vi "Abort Panel VI.vi"(8 "error in (no error)":errorcluster, 11 "Console in":refnum<class "Console.lvclass">) -> (0 "error out":errorcluster, 3 "Console out":refnum<class "Console.lvclass">)   [LabVIEW 2015, in "EditPanel API.lvlib" / "Console.lvclass"]
uses:
  Console.lvclass
  Console.lvclass/Console.ctl
  Console Reply/Console Reply/Console Reply.lvclass/Console Reply.ctl
  Console Reply/Console Reply/Console Reply.lvclass
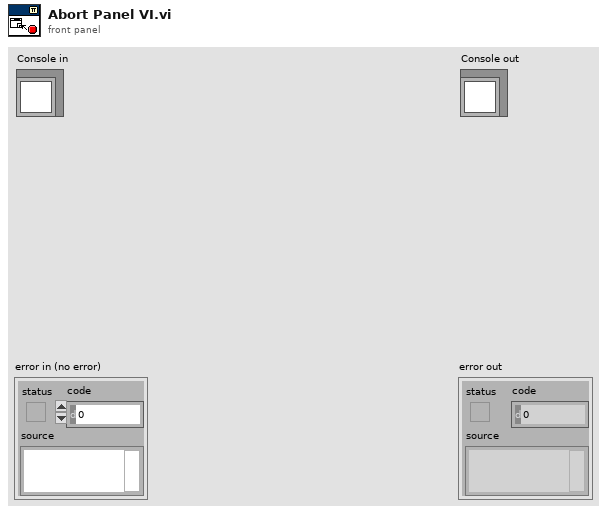
[diagram p1: front panel]
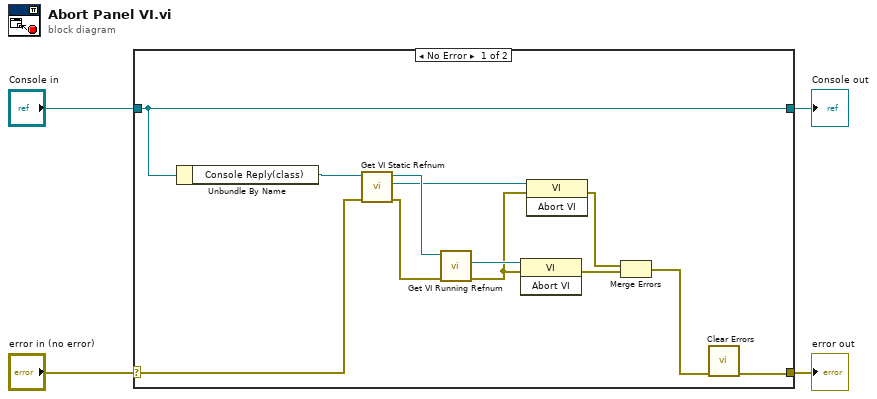
[diagram p0: block diagram]
diagram:
  n1 = case shown="No Error" "error in (no error)" {
    selector: "error in (no error)" -> [w13 w18]
    tunnel: [w15 w18] -> w3
    tunnel: [w16 w17] -> w1
    tunnel: "Console in" -> [w16 w17]
    frame No Error {
      n2 = Unbundle By Name(w16) -> ("Console Reply(class)"=w14:refnum<class "Console Reply.lvclass">)
      n3 = call "Get VI Static Refnum.vi"("error in (no error)"=w13, "Console Reply in"=w14) -> ("error out"=w11:errorcluster, "VI Static Refnum"=w9:refnum<vi>, "Console Reply out"=w12:refnum<class "Console Reply.lvclass">)  [unwired: 7 in]
      n4 = call "Get VI Running Refnum.vi"("error in (no error)"=w11, "Console Reply.lvclass"=w12) -> ("error out"=w6:errorcluster, "VI Running Refnum"=w7:refnum<vi>)  [unwired: 7 in, 1 out]
      n5 = invoke class="VI" method="Abort VI"(reference=w7, error in=w6) -> (error out=w5:errorcluster)  [unwired: 1 in, 2 out]
      n6 = invoke class="VI" method="Abort VI"(reference=w9, error in=w6) -> (error out=w8:errorcluster)  [unwired: 1 in, 2 out]
      n7 = Merge Errors(w8, w5) -> (w10:errorcluster)
      n8 = call <vilib>:"Clear Errors.vi"("error in (no error)"=w10) -> ("error out"=w15:errorcluster)  [unwired: 5 in, 1 out]
    }
    frame Error {
    }
  }
  "error out" <- w3
  "Console out" <- w1
